vi "create_file (SubVI).vi"(0 "Pulse Amplitude":dbl=1.4 format="%#_13g", 1 "Trigger Width (us)":dbl format="%#_13g", 4 "Frequency (MHz)":dbl, 5 "DAC frequency (MHz)":dbl, 6 "Numeric":i32, 7 "file path (use dialog)":path, 8 "Pulse Center":dbl format="%#_13g", 9 "Amplitude":dbl, 10 "Envelope Decay Time (micro s)":dbl, 11 "Number Of Points(integer multiple of 4096)":i32) -> (2 "output waveform 2":waveform(dbl)(graph), 3 "output waveform":waveform(dbl)(graph))   [LabVIEW 2016]
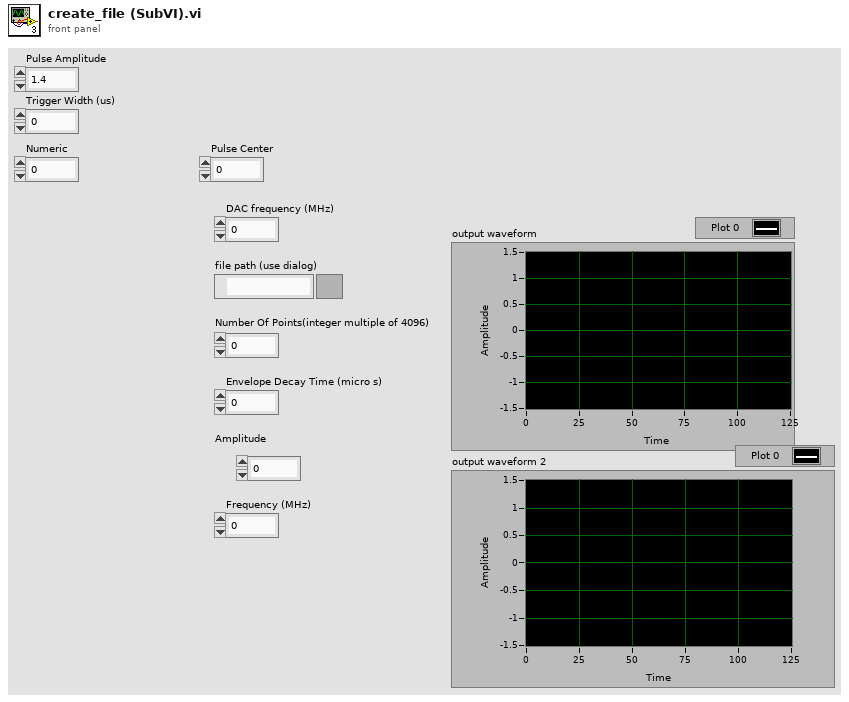
[diagram p1: front panel]
types:
  T1 = enum16{"open", "replace", "create", "open or create", "replace or create", "replace or create with confirmation"}
  T2 = enum16{"big-endian, network order", "native, host order", "little-endian"}
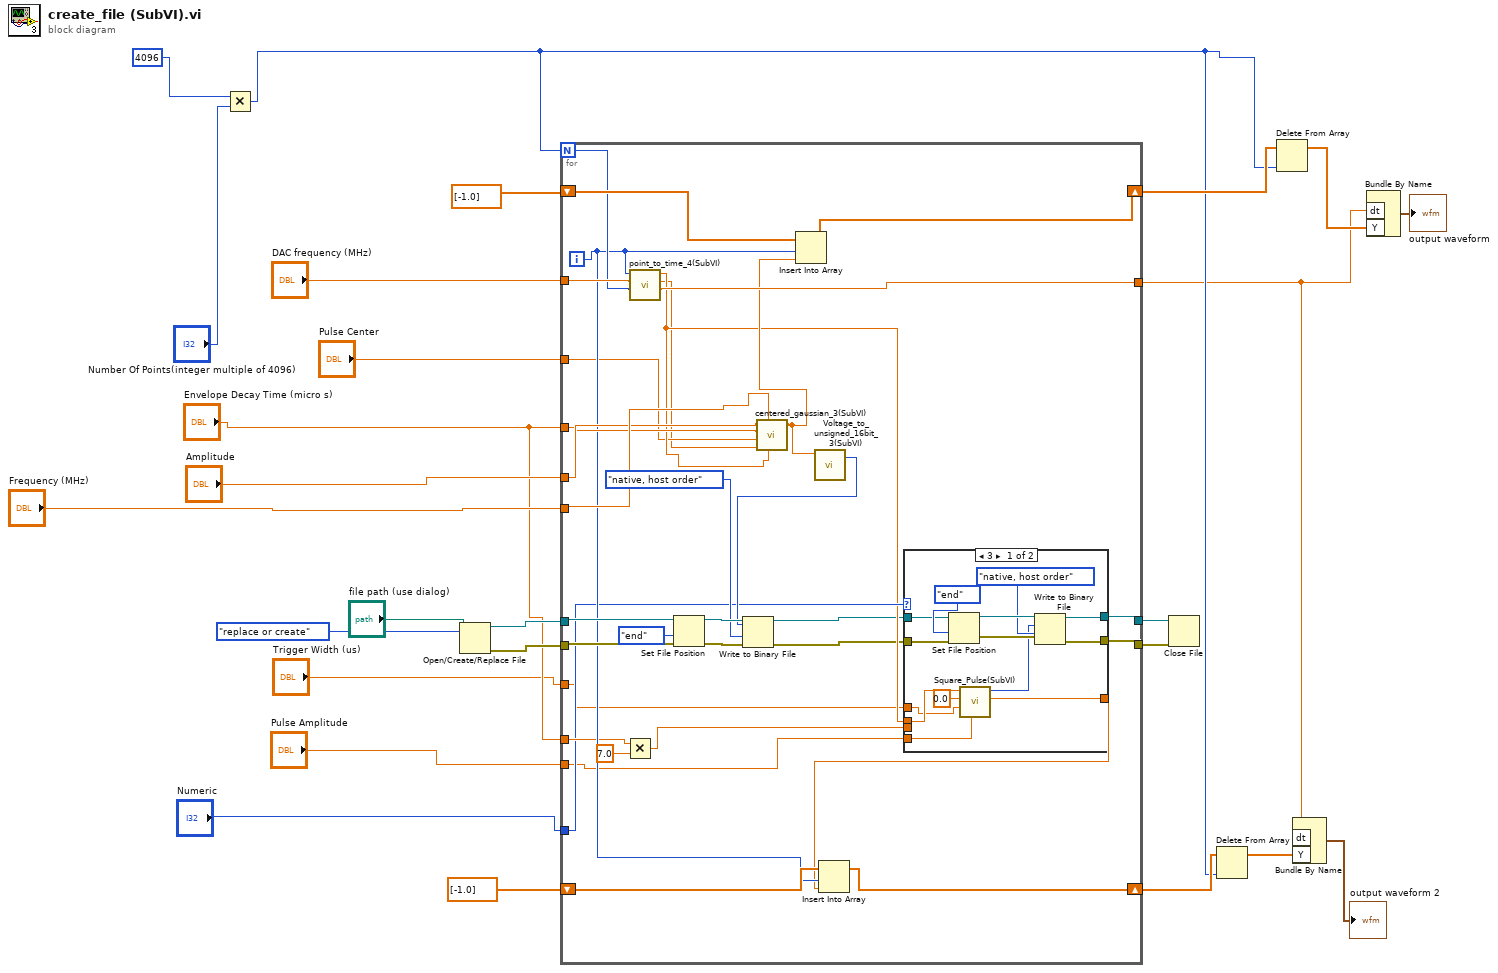
[diagram p0: block diagram]
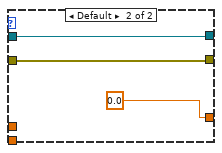
[diagram p2: hidden frame]
diagram:
  n1 = Multiply(x=4096, y="Number Of Points(integer multiple of 4096)") -> (x*y=w4:i32)
  n2 = Open/Create/Replace File(file path (use dialog)="file path (use dialog)", operation (0:open)=T1."replace or create") -> (refnum out=w22:refnum<file>, error out=w23:errorcluster)  [unwired: 4 in, 1 out]
  n3 = for {
    N: w4 -> [w49]
    tunnel: "Amplitude" -> [w45]
    shift-right: [w58] -> w26
    shift-left: dbl[] [-1.0] ("array") -> [w59]
    tunnel: "Envelope Decay Time (micro s)" -> [w44]
    tunnel: "Frequency (MHz)" -> [w47]
    tunnel: "DAC frequency (MHz)" -> [w50]
    tunnel: [w48] -> w3
    tunnel: w22 -> [w57]
    tunnel: w23 -> [w56]
    tunnel: [w31] -> w24
    tunnel: [w30] -> w25
    tunnel: "Pulse Center" -> [w34]
    tunnel: "Pulse Amplitude" -> [w37]
    tunnel: "Envelope Decay Time (micro s)" -> [w40]
    shift-right: [w41] -> w5
    shift-left: dbl[] [-1.0] ("array") -> [w43]
    tunnel: "Numeric" -> [w38]
    tunnel: "Trigger Width (us)" -> [w28]
    i -> [w42]
    n4 = Multiply(x=w40, y=7.0) -> (x*y=w33:dbl)
    n5 = call "point_to_time_4(SubVI).vi"("number of points"=w49, "DAC frequency(MHz)"=w50, "point location"=w42) -> ("dt (us)"=w48:dbl, "Pulse Width (us)"=w27:dbl, "time (us)"=w35:dbl)  [unwired: 6 in]
    n6 = Set File Position(refnum=w57, from (0:start)=enum16{"start", "end", "current"}."end", error in=w56) -> (refnum out=w55:refnum<file>, error out=w54:errorcluster)  [unwired: 1 in]
    n7 = call "centered_gaussian_3(SubVI).vi"("time"=w35, "Frequency(MHz)"=w47, "Pulse Lenth (us)"=w27, "Pulse Center"=w34, "Envelope DecayTime(micro s)"=w44, "Amplitude"=w45) -> ("output"=w46:dbl)  [unwired: 5 in]
    n8 = Insert Into Array(array=w59, index=w42, new element=w46) -> (w58:dbl[])
    n9 = call "Voltage_to_unsigned_16bit_3(SubVI).vi"("Voltage_in"=w46) -> ("unsigned 16bit integer"=w51:u16)  [unwired: 10 in]
    n10 = Write to Binary File(file (use dialog)=w55, data=w51, error in=w54, 9:T2."native, host order" ("byte order (0:big-endian, network order)")) -> (refnum out=w29:refnum<file>, error out=w32:errorcluster)  [unwired: 2 in, 1 out]
    n11 = case shown="3" w38 {
      tunnel: w37 -> [w73 _]
      tunnel: [w72 0.0] -> w36
      tunnel: w35 -> [w71 _]
      tunnel: w33 -> [_ _]
      tunnel: w32 -> [w69 w76]
      tunnel: [w66 w75] -> w31
      tunnel: [w65 w76] -> w30
      tunnel: w29 -> [w62 w75]
      tunnel: w28 -> [w60 _]
      frame 3 {
        n12 = Set File Position(refnum=w62, from (0:start)=enum16{"start", "end", "current"}."end", error in=w69) -> (refnum out=w68:refnum<file>, error out=w67:errorcluster)  [unwired: 1 in]
        n13 = call "Square_Pulse(SubVI).vi"("High Voltage (V)"=w73, "Pulse Width"=w60, "Pulse Start (us)"=0.0, "Time"=w71) -> ("Voltage Out"=w72:dbl, "unsigned 16-bit out"=w63:u16)  [unwired: 6 in]
        n14 = Write to Binary File(file (use dialog)=w68, data=w63, error in=w67, 9:T2."native, host order" ("byte order (0:big-endian, network order)")) -> (refnum out=w66:refnum<file>, error out=w65:errorcluster)  [unwired: 2 in, 1 out]
      }
      frame Default {
      }
    }
    n15 = Insert Into Array(array=w43, index=w42, new element=w36) -> (w41:dbl[])
  }
  n16 = Close File(refnum=w24, error in=w25) -> ()  [unwired: 2 out]
  n17 = Delete From Array(array=w5, index=w4) -> (array with subset deleted=w7:dbl[])  [unwired: 1 in, 1 out]
  n18 = Delete From Array(array=w26, index=w4) -> (array with subset deleted=w19:dbl[])  [unwired: 1 in, 1 out]
  n19 = Bundle By Name("dt"=w3, "Y"=w7) -> (→"output waveform 2":waveform(dbl))  [unwired: 1 in]
  n20 = Bundle By Name("dt"=w3, "Y"=w19) -> (→"output waveform":waveform(dbl))  [unwired: 1 in]
